vi "donut Animate.vi"() -> ()   [LabVIEW 2012]
doc: "This VI demonstrates how to animate a picture on the front panel using a picture ring (Pict Ring) control. This VI takes a sequence of pictures where each picture represents a \"frame\" of the animaction and makes each picture a selection in the picture ring. By programmatically incrementing the value of the picture ring, the picture appears to be animated."
uses:
  Rectangle Tools/Rect/Rect Tools.lvlib
panel:
  out "Pic Array":picture[](array[picture])
  in  "停止":bool
  in  "等待时间（毫秒）":u32=100
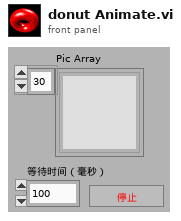
[diagram p1: front panel]
types:
  T1 = typedef "LVBoundsTypeDef.ctl" = cluster{"Width":u32, "Height":u32}
  T2 = cluster{"left":i16, "top":i16, "right":i16, "bottom":i16}
  T3 = typedef "imagedata.ctl" = cluster{"image type":i32, "image depth":i32, "image":u8[], "mask":u8[], "colors":u32[], "Rectangle":cluster{"left":i16, "top":i16, "right":i16, "bottom":i16}}
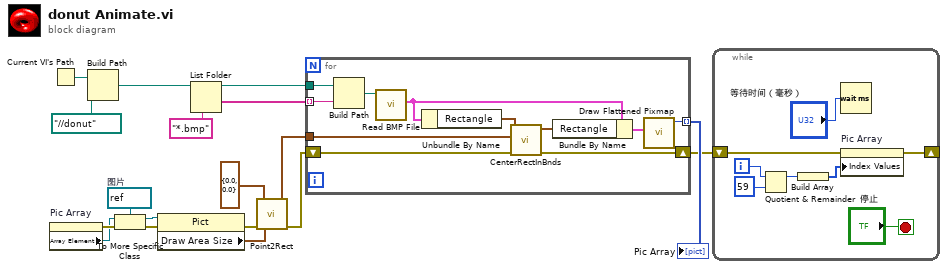
[diagram p0: block diagram]
diagram:
  w8 = refnum<vi> refnum  # 图片
  n1 = property on="Pic Array" class="Arr (严格)"() -> (error out=w10:errorcluster, "Array Element"=w9:refnum<vi>)  [unwired: 2 in, 1 out]
  n2 = Current VI's Path() -> (path=w17:path)
  n3 = Build Path(base path=w17, name or relative path=path "../../donut" ("基路径")) -> (appended path=w13:path)
  n4 = To More Specific Class(target class=w8, reference=w9, error in=w10) -> (specific class reference=w7:refnum<vi>, error out=w6:errorcluster)
  n5 = property class="Pict"(reference=w7, error in=w6) -> (error out=w4:errorcluster, "Draw Area Size"=w5:T1)  [unwired: 1 out]
  n6 = List Folder(path=w13, pattern="*.bmp" ("模式")) -> (path out=w1:path, filenames=w14:string[])  [unwired: 2 in, 2 out]
  n7 = call "Point2Rect.vi"("错误输入"=w4, "point b"=w5, "point a"=cluster{"x":dbl, "y":dbl} {"x"=0.0, "y"=0.0}) -> ("错误输出"=w3:errorcluster, "rect"=w12:T2)  [unwired: 7 in]
  n8 = for {
    tunnel: w14 -> [w28] mode=indexing
    tunnel: w1 -> [w29]
    tunnel: w12 -> [w27]
    tunnel: [w21] -> w11 mode=indexing
    shift-right: [w19] -> w2
    shift-left: w3 -> [w20]
    n9 = Build Path(base path=w29, name or relative path=w28) -> (appended path=w23:path)
    n10 = call <vilib>:"Read BMP File.vi"("path to BMP file"=w23) -> ("image data"=w26:T3)  [unwired: 8 in, 2 out]
    n11 = Unbundle By Name(w26) -> ("Rectangle"=w25:T2)
    n12 = call "CenterRectInBnds.vi"("错误输入"=w20, "bounds"=w27, "rect"=w25) -> ("错误输出"=w19:errorcluster, "centered rect"=w24:T2)  [unwired: 7 in]
    n13 = Bundle By Name(cluster=w26, "Rectangle"=w24) -> (w22:T3)
    n14 = call <vilib>:"Draw Flattened Pixmap.vi"("image data"=w22) -> ("new picture"=w21:picture)  [unwired: 8 in]
  }
  "Pic Array" <- w11
  n15 = while {
    shift-right: [w30] -> _
    shift-left: w2 -> [w31]
    i -> [w37]
    stop <- "停止" stop-if-true
    n16 = Quotient & Remainder(x=w37, y=59) -> (x-y*floor(x/y)=w33:i32)  [unwired: 1 out]
    n17 = Build Array(w33) -> (w32:i32[])
    n18 = Wait (ms)(milliseconds to wait="等待时间（毫秒）") -> ()  [unwired: 1 out]
    n19 = property on="Pic Array" class="Arr (严格)"(error in=w31, "Index Values"=w32) -> (error out=w30:errorcluster)  [unwired: 1 in, 1 out]
  }
